vi "reflexe-audio.vi"() -> (3 "reflexe (ms)":u32)   [LabVIEW 2025]
uses:
  <vilib>/numeric/Random Number (Range) U64.vi
  <vilib>/Analysis/baseanly.llb/Mean (DBL).vi
  <vilib>/numeric/sub_Random U32.vi
  <vilib>/Analysis/NI_AALBase.lvlib
panel:
  out "Waveform Graph 2":dbl[](graph)
  out "Waveform Graph":u32[](graph)
  out "Memoire":u32[](array[numeric])
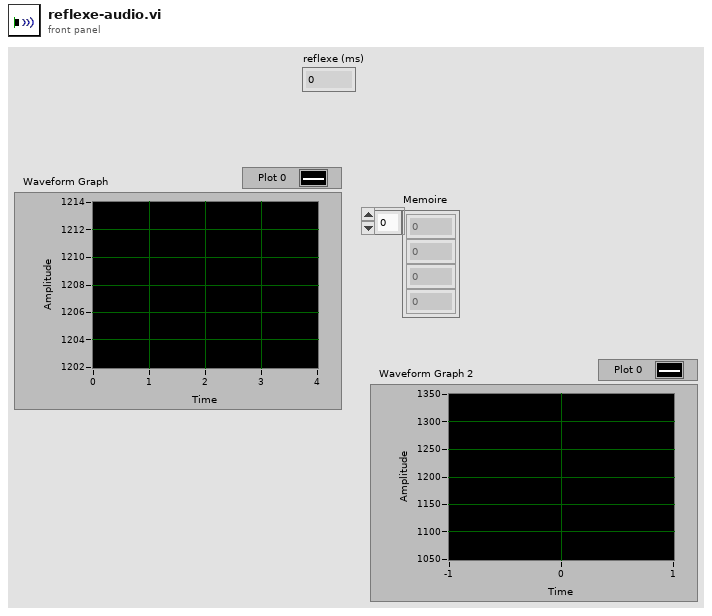
[diagram p1: front panel]
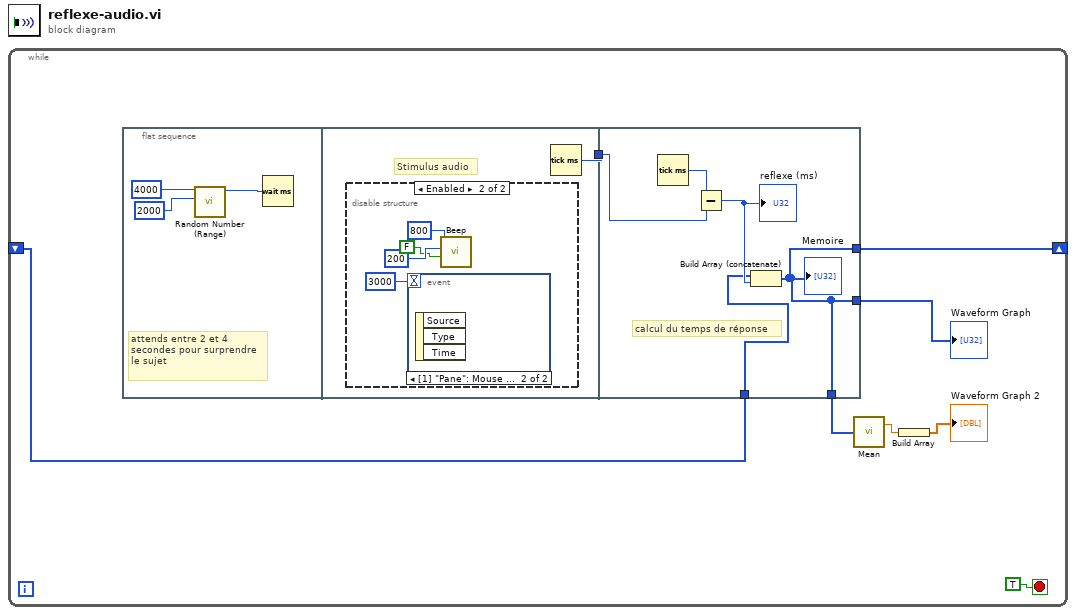
[diagram p0: block diagram]
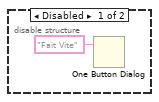
[diagram p2: hidden frame]
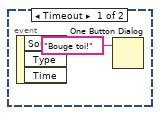
[diagram p3: hidden frame]
diagram:
  n1 = while {
    shift-right: [w6] -> _
    shift-left: _ -> [w5]
    stop <- TRUE stop-if-true
    n2 = flat-sequence {
      tunnel: [w12] -> w7
      tunnel: w7 -> [w22]
      tunnel: [w19] -> w6
      tunnel: w5 -> [w20]
      tunnel: [w19] -> w4
      tunnel: [w19] -> w3
      frame #0 {
        # "attends entre 2 et 4 secondes pour surprendre le sujet"
        n3 = call-poly <vilib>:"Random Number (Range).vi"("lower bound (0)"=u64 2000, "upper bound (100)"=u64 4000) -> ("number"=w11:u64)  [unwired: 9 in]
        n4 = Wait (ms)(milliseconds to wait=w11) -> ()  [unwired: 1 out]
      }
      frame #1 {
        # "Stimulus audio"
        n5 = disable-structure shown="Enabled" {
          frame Disabled {
            n6 = One Button Dialog(message="Fait Vite") -> ()  [unwired: 1 in, 1 out]
          }
          frame Enabled {
            n7 = event shown="[1] \"Pane\": Mouse Down" {
              selector: _ -> [_ _]
              dyn-events: _ -> [_ _]
              timeout: 3000 -> [_ _]
              event Timeout {
                n8 = event-data() -> ()  [unwired: 1 in, 3 out]
                n9 = One Button Dialog(message="Bouge toi!") -> ()  [unwired: 1 in, 1 out]
              }
              event Mouse Down {
                n10 = event-data() -> ()  [unwired: 1 in, 3 out]
              }
            }
            n11 = call <vilib>:"Beep.vi"("use system alert? (T)"=FALSE, "duration (msec)"=u32 200, "frequency (Hz)"=u32 800) -> ()  [unwired: 9 in]
          }
        }
        n12 = Tick Count (ms)() -> (millisecond timer value=w12:u32)
      }
      frame #2 {
        # "calcul du temps de réponse"
        n13 = Tick Count (ms)() -> (millisecond timer value=w23:u32)
        n14 = Subtract(x=w23, y=w22) -> (x-y=w21:u32)
        "reflexe (ms)" <- w21
        n15 = Build Array (concatenate)(w20, w21) -> (w19:u32[])
        "Memoire" <- w19
      }
    }
    n16 = call-poly <vilib>:"Mean.vi"("X"=w3) -> ("mean"=w2:dbl)  [unwired: 1 out]
    n17 = Build Array(w2) -> (→"Waveform Graph 2":dbl[])
    "Waveform Graph" <- w4
  }
